vi "Shooting.vi"(11 "input cluster":T1) -> ()   [LabVIEW 2015]
uses:
  Joystick/ControlsToCommands.ctl
  Robot Global Data.vi
  References/Refnums.vi
  <vilib>/Rock Robotics/Network Tables/NT Write String.vi
panel:
  out "SpeeD":dbl=0.8
  in  "Speed 2":dbl
  in  "Speed1":dbl
  in  "Manual Shoot":bool
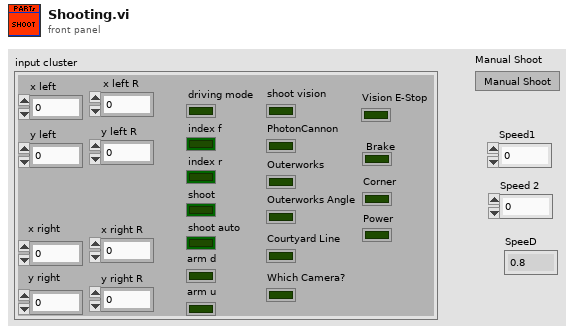
[diagram p1: front panel]
types:
  T1 = typedef "ControlsToCommands.ctl" = cluster{"x left":dbl, "y left":dbl, "x right":dbl, "y right":dbl, "driving mode":bool, "index f":bool, "index r":bool, "shoot":bool, "shoot auto":bool, "arm d":bool, "arm u":bool, "shoot vision":bool, "PhotonCannon":bool, "Outerworks":bool, "Outerworks Angle":bool, "Courtyard Line":bool, "Which Camera?":bool, "Vision E-Stop":bool, "x left R":dbl, "y left R":dbl, "x right R":dbl, "y right R":dbl, "Brake":bool, "Corner":bool, "Power":bool}
  T2 = typedef "WPI_MotorControlDeviceRef.ctl" = cluster{"DeviceStatus":errorcluster, "Type":T3, "PWM":cluster{"PWM Channel":T4, "DeadBand":T5}, "CAN":cluster{"Device Number":u8, "Control Mode":T6, "Semaphore":T7, "Max Vout":dbl, "TalonSRX Control Mode":T8}, "Invert":bool}
  T3 = typedef "WPI_MotorControlType.ctl" = enum16{"PWM", "CAN", "CANTalonSRX"}
  T4 = typedef "FPGA_DIOPWMChannel.ctl" = enum8{"PWM 0", "PWM 1", "PWM 2", "PWM 3", "PWM 4", "PWM 5", "PWM 6", "PWM 7", "PWM 8", "PWM 9", "PWM MXP 0", "PWM MXP 1", "PWM MXP 2", "PWM MXP 3", "PWM MXP 4", "PWM MXP 5", "PWM MXP 6", "PWM MXP 7", "PWM MXP 8", "PWM MXP 9", "Invalid"}
  T5 = typedef "WPI_PWMDeadband.ctl" = cluster{"Name":string, "maxPositivePwm":i32, "minPositivePwm":i32, "centerPwm":i32, "maxNegativePwm":i32, "minNegativePwm":i32, "angularRange":u16}
  T6 = typedef "WPI_CANJaguar_ControlMode.ctl" = enum8{"Percent VBus", "Current", "Speed", "Position", "Voltage"}
  T7 = typedef "Semaphore RefNum" = refnum<k1>
  T8 = typedef "WPI_CANTalonSRX_APIControlMode.ctl" = enum8{"Percent VBus", "Speed", "Position", "Slave", "Unchanged / Invalid", "Voltage Compensation", "Current", "Motion Profile"}
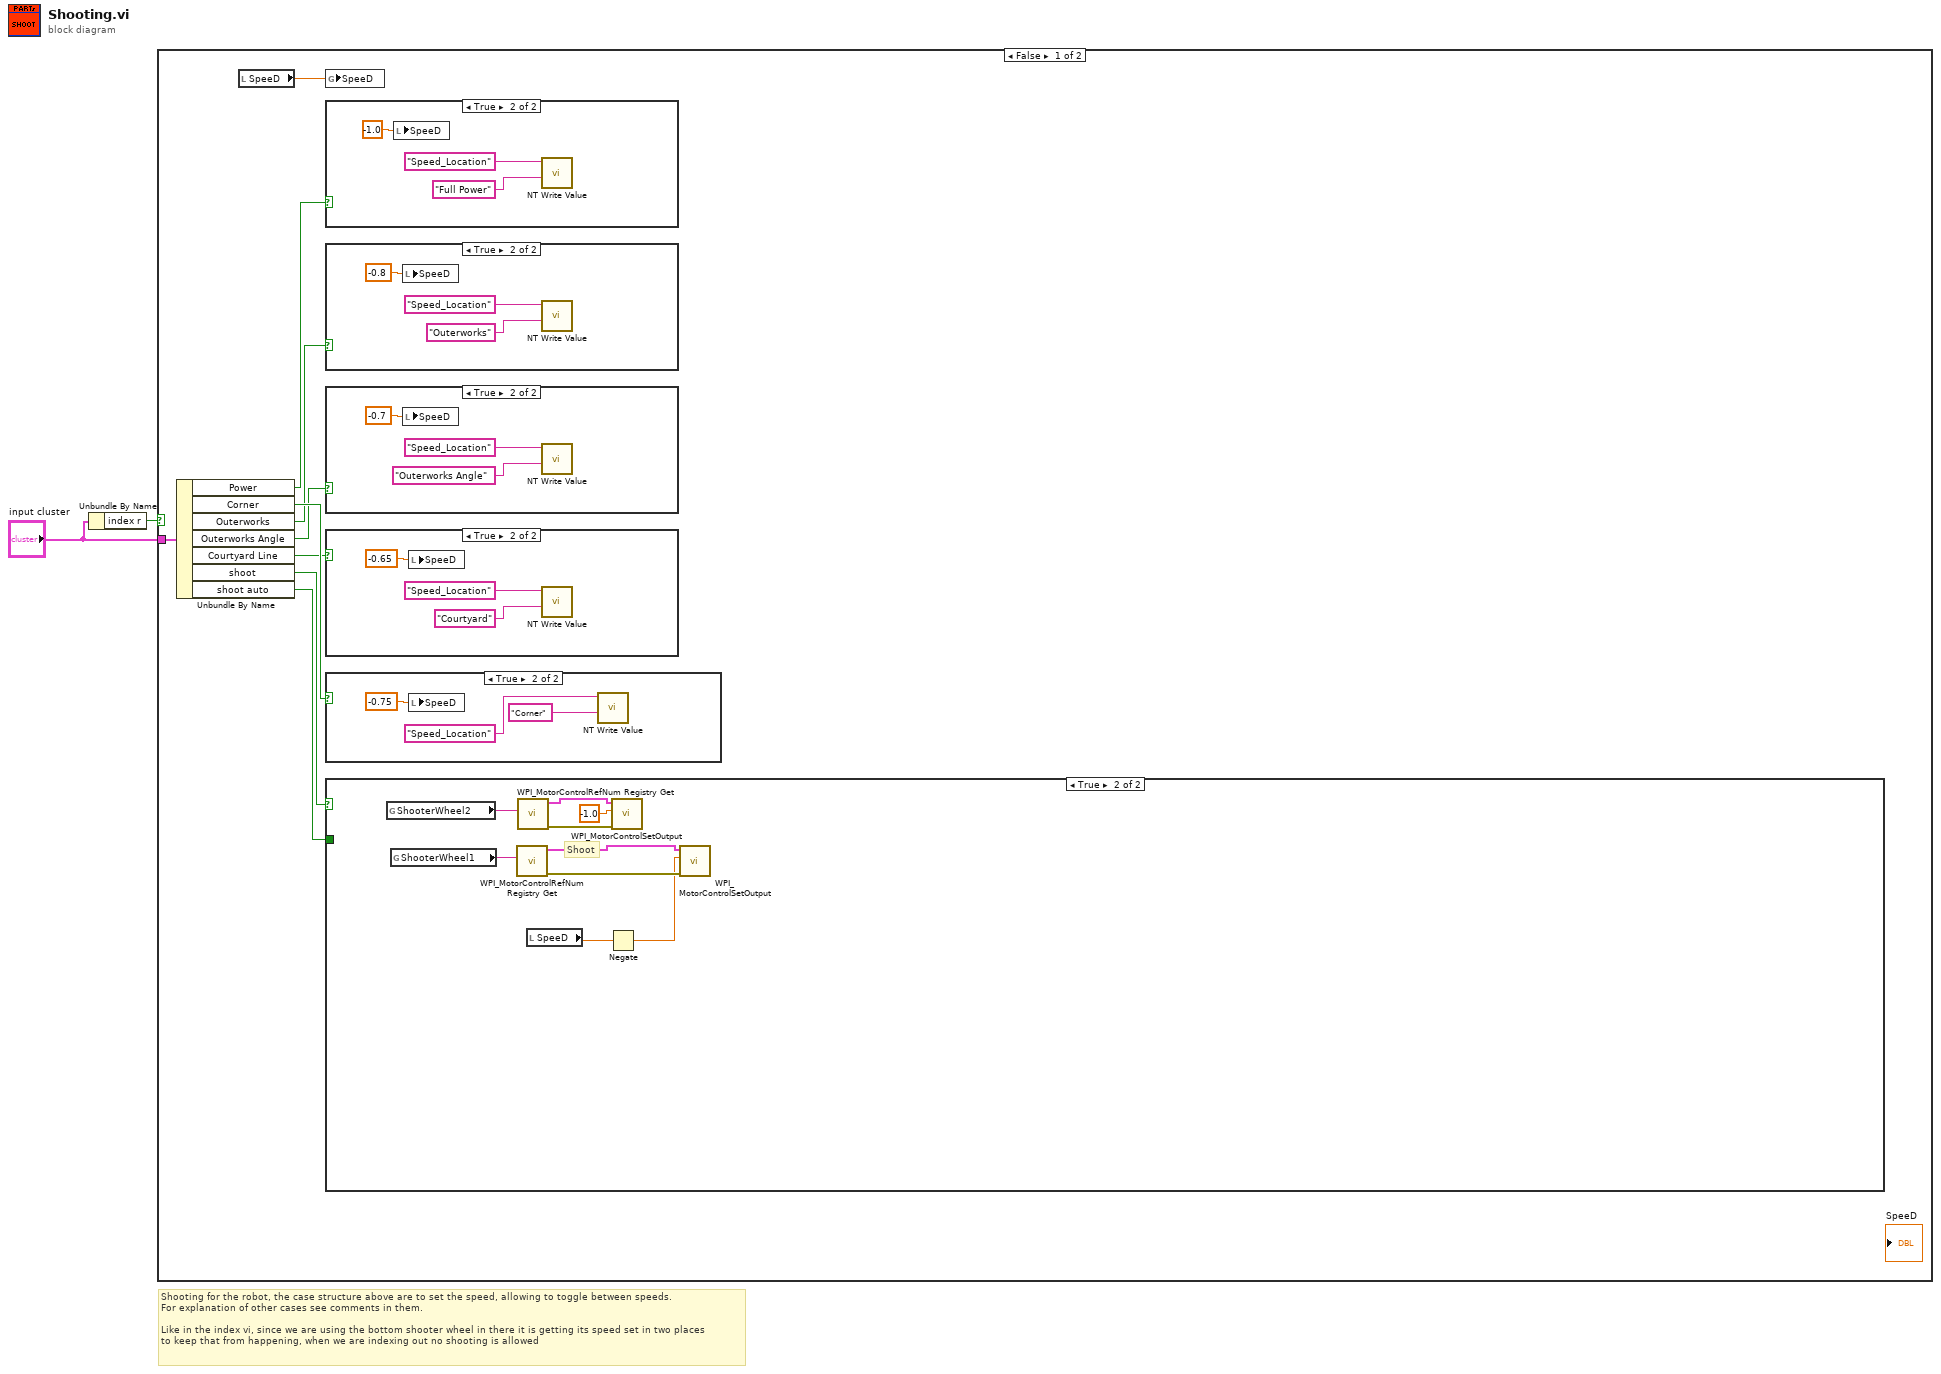
[diagram p0: block diagram]
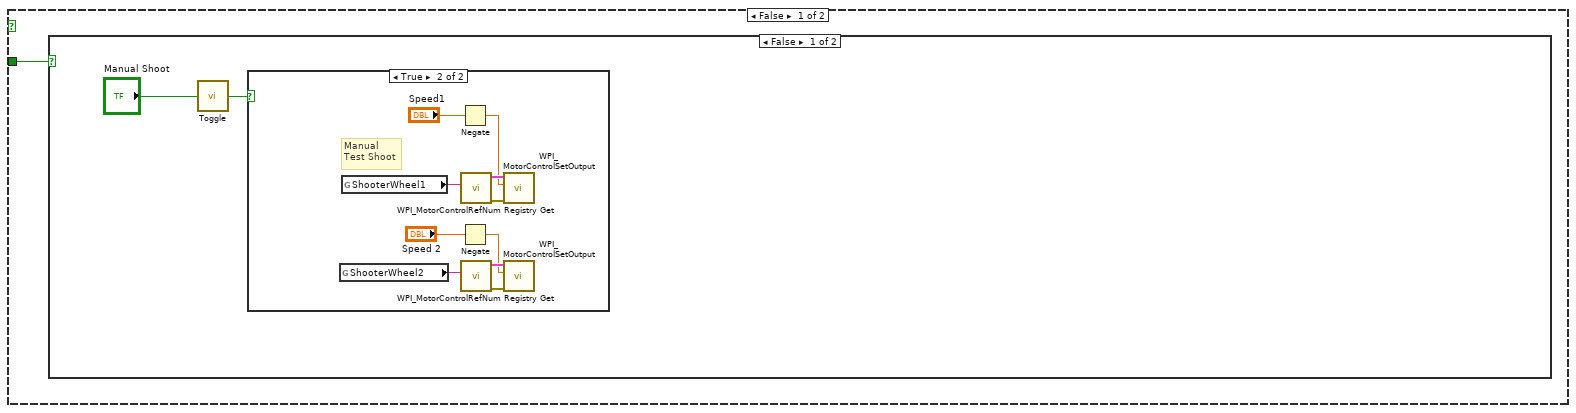
[diagram p7: hidden frame]
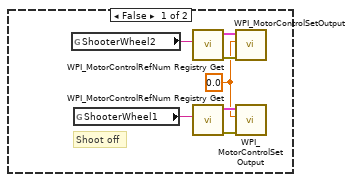
[diagram p8: hidden frame]
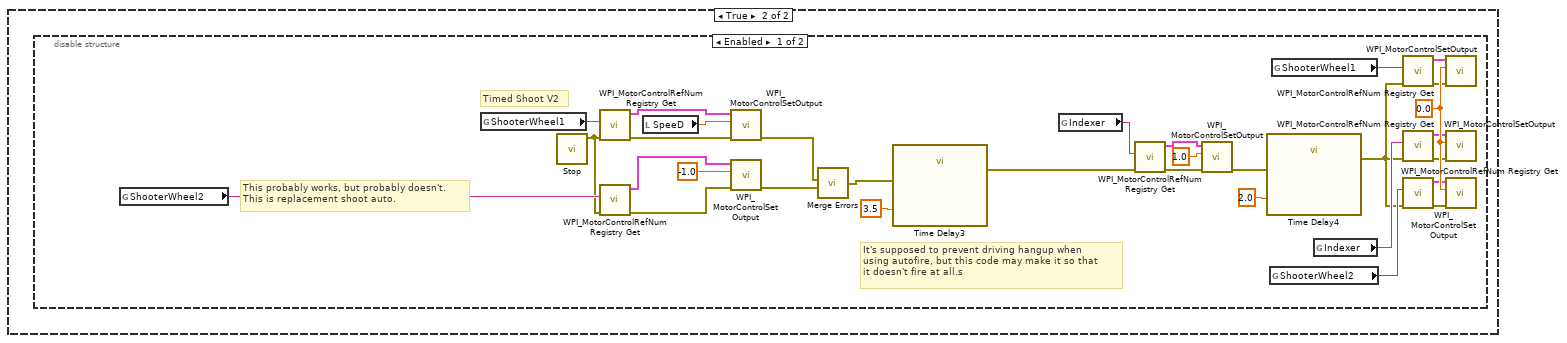
[diagram p9: hidden frame]
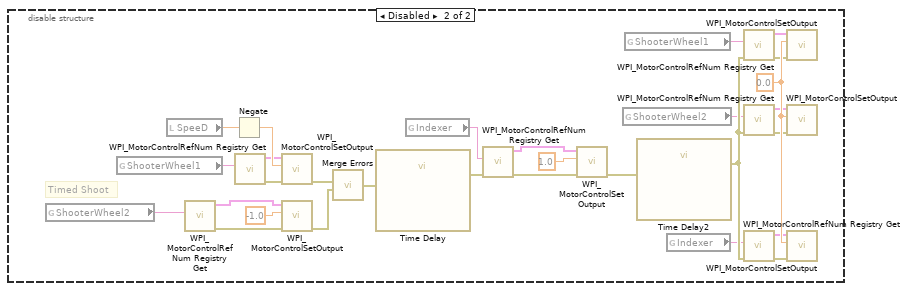
[diagram p10: hidden frame]
diagram:
  # "Shooting for the robot, the case structure above are to set the speed, allowing to toggle between speeds. \nFor explanation of other cases see comments in them.\n\nLike in the index vi, since we are using the bottom shooter wheel in there it is getting its speed set in two places\nto keep that from happening, when we are indexing out no shooting is allowed"
  n1 = Unbundle By Name("input cluster") -> ("index r"=w1:bool)
  n2 = case shown="False" w1 {
    tunnel: "input cluster" -> [w11 _]
    frame False {
      n3 = Unbundle By Name(w11) -> ("Power"=w3:bool, "Corner"=w9:bool, "Outerworks"=w8:bool, "Outerworks Angle"=w7:bool, "Courtyard Line"=w6:bool, "shoot"=w5:bool, "shoot auto"=w4:bool)
      n4 = local read "SpeeD"() -> (w10:dbl)
      n5 = global write "Robot Global Data.vi" "SpeeD"(w10) -> ()
      n6 = case shown="True" w3 {
        frame False {
        }
        frame True {
          n7 = local write "SpeeD"(-1.0) -> ()
          n8 = call-poly <vilib>:"NT Write Value.vi"("String"="Full Power", "Name"="Speed_Location") -> ()  [unwired: 9 in, 1 out]
        }
      }
      n9 = case shown="True" w8 {
        frame False {
        }
        frame True {
          n10 = local write "SpeeD"(-0.8) -> ()
          n11 = call-poly <vilib>:"NT Write Value.vi"("String"="Outerworks", "Name"="Speed_Location") -> ()  [unwired: 9 in, 1 out]
        }
      }
      n12 = case shown="True" w7 {
        frame False {
        }
        frame True {
          n13 = local write "SpeeD"(-0.7) -> ()
          n14 = call-poly <vilib>:"NT Write Value.vi"("String"="Outerworks Angle", "Name"="Speed_Location") -> ()  [unwired: 9 in, 1 out]
        }
      }
      n15 = case shown="True" w6 {
        frame False {
        }
        frame True {
          n16 = local write "SpeeD"(-0.65) -> ()
          n17 = call-poly <vilib>:"NT Write Value.vi"("String"="Courtyard", "Name"="Speed_Location") -> ()  [unwired: 9 in, 1 out]
        }
      }
      n18 = case shown="True" w9 {
        frame False {
        }
        frame True {
          n19 = local write "SpeeD"(-0.75) -> ()
          n20 = call-poly <vilib>:"NT Write Value.vi"("String"="Corner", "Name"="Speed_Location") -> ()  [unwired: 9 in, 1 out]
        }
      }
      n21 = case shown="True" w5 {
        tunnel: w4 -> [w27 _]
        frame False {
          n22 = case shown="False" w27 {
            frame False {
              n23 = call "Toggle.vi"("Input"="Manual Shoot") -> ("Output"=w28:bool)  [unwired: 4 in]
              n24 = case shown="True" w28 {
                frame False {
                  w30 = 0.0 ("Output")
                  # "Shoot off"
                  n25 = global read "Refnums.vi" "ShooterWheel2"() -> (w34:string)
                  n26 = global read "Refnums.vi" "ShooterWheel1"() -> (w33:string)
                  n27 = call <vilib>:"WPI_MotorControlRefNum Registry Get.vi"("refnum name"=w34) -> ("error out"=w35:errorcluster, "MotorControlDevRef"=w36:T2)  [unwired: 9 in]
                  n28 = call <vilib>:"WPI_MotorControlRefNum Registry Get.vi"("refnum name"=w33) -> ("error out"=w31:errorcluster, "MotorControlDevRef"=w32:T2)  [unwired: 9 in]
                  n29 = call <vilib>:"WPI_MotorControlSetOutput.vi"("error in (no error)"=w35, "Output"=w30, "MotorControlDevRef"=w36) -> ()  [unwired: 6 in, 3 out]
                  n30 = call <vilib>:"WPI_MotorControlSetOutput.vi"("error in (no error)"=w31, "Output"=w30, "MotorControlDevRef"=w32) -> ()  [unwired: 6 in, 3 out]
                }
                frame True {
                  # "Manual\nTest Shoot"
                  n31 = global read "Refnums.vi" "ShooterWheel2"() -> (w44:string)
                  n32 = global read "Refnums.vi" "ShooterWheel1"() -> (w43:string)
                  n33 = Negate(x="Speed1") -> (-x=w40:dbl)
                  n34 = Negate(x="Speed 2") -> (-x=w37:dbl)
                  n35 = call <vilib>:"WPI_MotorControlRefNum Registry Get.vi"("refnum name"=w43) -> ("error out"=w41:errorcluster, "MotorControlDevRef"=w42:T2)  [unwired: 9 in]
                  n36 = call <vilib>:"WPI_MotorControlRefNum Registry Get.vi"("refnum name"=w44) -> ("error out"=w45:errorcluster, "MotorControlDevRef"=w46:T2)  [unwired: 9 in]
                  n37 = call <vilib>:"WPI_MotorControlSetOutput.vi"("error in (no error)"=w41, "Output"=w40, "MotorControlDevRef"=w42) -> ()  [unwired: 6 in, 3 out]
                  n38 = call <vilib>:"WPI_MotorControlSetOutput.vi"("error in (no error)"=w45, "Output"=w37, "MotorControlDevRef"=w46) -> ()  [unwired: 6 in, 3 out]
                }
              }
            }
            frame True {
              n39 = disable-structure shown="Enabled" {
                frame Enabled {
                  w68 = 0.0
                  # "Timed Shoot V2"
                  # "It's supposed to prevent driving hangup when \nusing autofire, but this code may make it so that \nit doesn't fire at all.s"
                  # "This probably works, but probably doesn't.\nThis is replacement shoot auto."
                  n40 = global read "Refnums.vi" "ShooterWheel2"() -> (w71:string)
                  n41 = global read "Refnums.vi" "ShooterWheel1"() -> (w72:string)
                  n42 = call "Stop.vi"() -> ("error out"=w47:errorcluster)  [unwired: 10 in, 1 out]
                  n43 = call <vilib>:"WPI_MotorControlRefNum Registry Get.vi"("error in (no error)"=w47, "refnum name"=w72) -> ("error out"=w74:errorcluster, "MotorControlDevRef"=w73:T2)  [unwired: 8 in]
                  n44 = call <vilib>:"WPI_MotorControlRefNum Registry Get.vi"("error in (no error)"=w47, "refnum name"=w71) -> ("error out"=w70:errorcluster, "MotorControlDevRef"=w69:T2)  [unwired: 8 in]
                  n45 = local read "SpeeD"() -> (w48:dbl)
                  n46 = call <vilib>:"WPI_MotorControlSetOutput.vi"("error in (no error)"=w74, "Output"=w48, "MotorControlDevRef"=w73) -> ("error out"=w76:errorcluster)  [unwired: 6 in, 2 out]
                  n47 = call <vilib>:"WPI_MotorControlSetOutput.vi"("error in (no error)"=w70, "Output"=-1.0, "MotorControlDevRef"=w69) -> ("error out"=w77:errorcluster)  [unwired: 6 in, 2 out]
                  n48 = call "Merge Errors.vi"("error in 2"=w77, "error in"=w76) -> ("error out"=w53:errorcluster)  [unwired: 2 in]
                  n49 = call "Time Delay3"("error in (no error)"=w53, "Delay Time (s)"=3.5) -> ("error out"=w52:errorcluster)  [unwired: 9 in]
                  n50 = global read "Refnums.vi" "Indexer"() -> (w58:string)
                  n51 = call <vilib>:"WPI_MotorControlRefNum Registry Get.vi"("error in (no error)"=w52, "refnum name"=w58) -> ("error out"=w56:errorcluster, "MotorControlDevRef"=w57:T2)  [unwired: 8 in]
                  n52 = call <vilib>:"WPI_MotorControlSetOutput.vi"("error in (no error)"=w56, "Output"=1.0, "MotorControlDevRef"=w57) -> ("error out"=w50:errorcluster)  [unwired: 6 in, 2 out]
                  n53 = call "Time Delay4"("error in (no error)"=w50, "Delay Time (s)"=2.0) -> ("error out"=w49:errorcluster)  [unwired: 9 in]
                  n54 = global read "Refnums.vi" "ShooterWheel2"() -> (w59:string)
                  n55 = global read "Refnums.vi" "ShooterWheel1"() -> (w60:string)
                  n56 = global read "Refnums.vi" "Indexer"() -> (w67:string)
                  n57 = call <vilib>:"WPI_MotorControlRefNum Registry Get.vi"("error in (no error)"=w49, "refnum name"=w60) -> ("error out"=w64:errorcluster, "MotorControlDevRef"=w63:T2)  [unwired: 8 in]
                  n58 = call <vilib>:"WPI_MotorControlRefNum Registry Get.vi"("error in (no error)"=w49, "refnum name"=w67) -> ("error out"=w65:errorcluster, "MotorControlDevRef"=w66:T2)  [unwired: 8 in]
                  n59 = call <vilib>:"WPI_MotorControlRefNum Registry Get.vi"("error in (no error)"=w49, "refnum name"=w59) -> ("error out"=w62:errorcluster, "MotorControlDevRef"=w61:T2)  [unwired: 8 in]
                  n60 = call <vilib>:"WPI_MotorControlSetOutput.vi"("error in (no error)"=w64, "Output"=w68, "MotorControlDevRef"=w63) -> ()  [unwired: 6 in, 3 out]
                  n61 = call <vilib>:"WPI_MotorControlSetOutput.vi"("error in (no error)"=w65, "Output"=w68, "MotorControlDevRef"=w66) -> ()  [unwired: 6 in, 3 out]
                  n62 = call <vilib>:"WPI_MotorControlSetOutput.vi"("error in (no error)"=w62, "Output"=w68, "MotorControlDevRef"=w61) -> ()  [unwired: 6 in, 3 out]
                }
                frame Disabled {
                  w103 = 0.0
                  # "Timed Shoot"
                  n63 = global read "Refnums.vi" "ShooterWheel2"() -> (w80:string)
                  n64 = global read "Refnums.vi" "ShooterWheel1"() -> (w81:string)
                  n65 = local read "SpeeD"() -> (w106:dbl)
                  n66 = call <vilib>:"WPI_MotorControlRefNum Registry Get.vi"("refnum name"=w80) -> ("error out"=w79:errorcluster, "MotorControlDevRef"=w78:T2)  [unwired: 9 in]
                  n67 = Negate(x=w106) -> (-x=w105:dbl)
                  n68 = call <vilib>:"WPI_MotorControlRefNum Registry Get.vi"("refnum name"=w81) -> ("error out"=w83:errorcluster, "MotorControlDevRef"=w82:T2)  [unwired: 9 in]
                  n69 = call <vilib>:"WPI_MotorControlSetOutput.vi"("error in (no error)"=w83, "Output"=w105, "MotorControlDevRef"=w82) -> ("error out"=w85:errorcluster)  [unwired: 6 in, 2 out]
                  n70 = call <vilib>:"WPI_MotorControlSetOutput.vi"("error in (no error)"=w79, "Output"=-1.0, "MotorControlDevRef"=w78) -> ("error out"=w86:errorcluster)  [unwired: 6 in, 2 out]
                  n71 = call "Merge Errors.vi"("error in 2"=w86, "error in"=w85) -> ("error out"=w87:errorcluster)  [unwired: 2 in]
                  n72 = call "Time Delay"("error in (no error)"=w87) -> ("error out"=w91:errorcluster)  [unwired: 10 in]
                  n73 = global read "Refnums.vi" "Indexer"() -> (w90:string)
                  n74 = call <vilib>:"WPI_MotorControlRefNum Registry Get.vi"("error in (no error)"=w91, "refnum name"=w90) -> ("error out"=w88:errorcluster, "MotorControlDevRef"=w89:T2)  [unwired: 8 in]
                  n75 = call <vilib>:"WPI_MotorControlSetOutput.vi"("error in (no error)"=w88, "Output"=1.0, "MotorControlDevRef"=w89) -> ("error out"=w93:errorcluster)  [unwired: 6 in, 2 out]
                  n76 = global read "Refnums.vi" "ShooterWheel2"() -> (w96:string)
                  n77 = global read "Refnums.vi" "ShooterWheel1"() -> (w97:string)
                  n78 = call "Time Delay2"("error in (no error)"=w93) -> ("error out"=w104:errorcluster)  [unwired: 10 in]
                  n79 = global read "Refnums.vi" "Indexer"() -> (w102:string)
                  n80 = call <vilib>:"WPI_MotorControlRefNum Registry Get.vi"("error in (no error)"=w104, "refnum name"=w97) -> ("error out"=w99:errorcluster, "MotorControlDevRef"=w98:T2)  [unwired: 8 in]
                  n81 = call <vilib>:"WPI_MotorControlRefNum Registry Get.vi"("error in (no error)"=w104, "refnum name"=w96) -> ("error out"=w95:errorcluster, "MotorControlDevRef"=w94:T2)  [unwired: 8 in]
                  n82 = call <vilib>:"WPI_MotorControlRefNum Registry Get.vi"("error in (no error)"=w104, "refnum name"=w102) -> ("error out"=w100:errorcluster, "MotorControlDevRef"=w101:T2)  [unwired: 8 in]
                  n83 = call <vilib>:"WPI_MotorControlSetOutput.vi"("error in (no error)"=w99, "Output"=w103, "MotorControlDevRef"=w98) -> ()  [unwired: 6 in, 3 out]
                  n84 = call <vilib>:"WPI_MotorControlSetOutput.vi"("error in (no error)"=w95, "Output"=w103, "MotorControlDevRef"=w94) -> ()  [unwired: 6 in, 3 out]
                  n85 = call <vilib>:"WPI_MotorControlSetOutput.vi"("error in (no error)"=w100, "Output"=w103, "MotorControlDevRef"=w101) -> ()  [unwired: 6 in, 3 out]
                }
              }
            }
          }
        }
        frame True {
          # "Shoot"
          n86 = global read "Refnums.vi" "ShooterWheel2"() -> (w111:string)
          n87 = global read "Refnums.vi" "ShooterWheel1"() -> (w112:string)
          n88 = call <vilib>:"WPI_MotorControlRefNum Registry Get.vi"("refnum name"=w112) -> ("error out"=w114:errorcluster, "MotorControlDevRef"=w113:T2)  [unwired: 9 in]
          n89 = call <vilib>:"WPI_MotorControlRefNum Registry Get.vi"("refnum name"=w111) -> ("error out"=w110:errorcluster, "MotorControlDevRef"=w109:T2)  [unwired: 9 in]
          n90 = local read "SpeeD"() -> (w108:dbl)
          n91 = Negate(x=w108) -> (-x=w107:dbl)
          n92 = call <vilib>:"WPI_MotorControlSetOutput.vi"("error in (no error)"=w110, "Output"=-1.0, "MotorControlDevRef"=w109) -> ()  [unwired: 6 in, 3 out]
          n93 = call <vilib>:"WPI_MotorControlSetOutput.vi"("error in (no error)"=w114, "Output"=w107, "MotorControlDevRef"=w113) -> ()  [unwired: 6 in, 3 out]
        }
      }
    }
    frame True {
    }
  }
